vi "end.vi"   [LabVIEW 2023]
types:
  T1 = enum16{"Initialize", "Absolute Position", "Relative Pickup", "Relative Dispense", "Swich valve", "Bypass"}
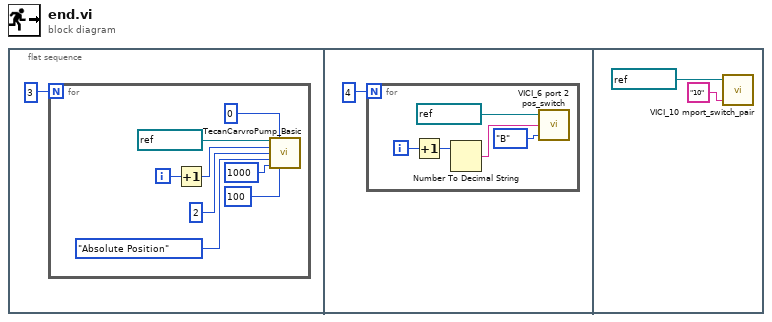
[diagram p0: block diagram]
diagram:
  n1 = flat-sequence {
    frame #0 {
      n2 = for {
        N: 3 -> [_]
        i -> [w3]
        n3 = Increment(x=w3) -> (x+1=w2:i32)
        n4 = call "TecanCarvroPump_Basic.vi"("TecanPump COM"=refnum<visa-resource-name> "COM6", "Volume (μL)"=u16 0, "TecanPump address"=w2, "Valve"=u8 2, "Mode"=T1."Absolute Position", "Syringe size (μL)"=u16 1000, "Speed (μL/s)"=u16 100) -> ()  [unwired: 8 in, 1 out]
      }
    }
    frame #1 {
      n5 = for {
        N: 4 -> [_]
        i -> [w15]
        n6 = Increment(x=w15) -> (x+1=w14:i32)
        n7 = Number To Decimal String(number=w14) -> (decimal integer string=w13:string)  [unwired: 1 in]
        n8 = call "VICI_6 port 2 pos_switch.vi"("Switch to position (A/B)"=enum16{"A", "B"}."B", "Valve ID"=w13, "Valve COM"=refnum<visa-resource-name> "COM8") -> ()  [unwired: 1 in, 1 out]
      }
    }
    frame #2 {
      n9 = call "VICI_10 mport_switch_pair.vi"("Go to position"="10", "Valve COM"=refnum<visa-resource-name> "COM8") -> ()  [unwired: 2 in, 1 out]
    }
  }
